vi "DAQmx Control Task.vi"(0 "task/channels in":refnum<k21>, 5 "action":i32(ring)=2 items=["verify"=2, "reserve"=4, "commit"=3, "unreserve"=5, "abort"=6], 11 "error in":errorcluster) -> (4 "task out":refnum<k21>, 15 "error out":errorcluster)   [LabVIEW 2020]
doc: "Alters the state of a task according to the <B>action</B> you specify."
uses:
  nilvaiu.dll
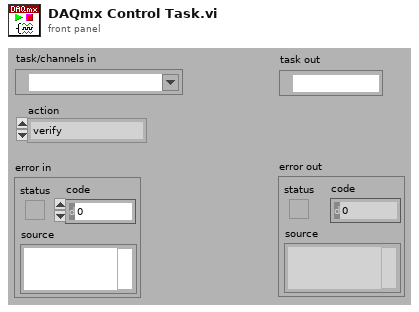
[diagram p1: front panel]
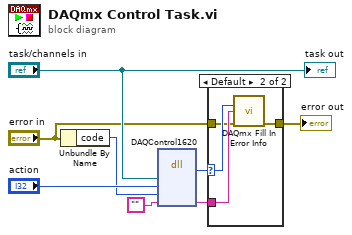
[diagram p0: block diagram]
diagram:
  n1 = Unbundle By Name("error in") -> ("code"=w1:i32)
  n2 = dll-call lib="nilvaiu.*" fn="DAQControl1620"("taskID"="task/channels in", "mode"="action", "incomingStatus"=w1, "extendedErrorInfo"="") -> ("return type"=w4:i32, "extendedErrorInfo"=w5:string)  [unwired: 5 in, 3 out]
  n3 = case shown="Default" w4 {
    selector: w4 -> [_ w12]
    tunnel: [w9 w13] -> w7
    tunnel: w5 -> [_ w11]
    tunnel: "error in" -> [w9 w10]
    frame 0 {
    }
    frame Default {
      n4 = call "DAQmx Fill In Error Info.vi"("status code"=w12, "extended error info"=w11, "error in"=w10) -> ("error out"=w13:errorcluster)  [unwired: 1 in, 11 out]
    }
  }
  "error out" <- w7
  "task out" <- "task/channels in"
